vi "Deliver Result.vi"(8 "error in (no error)":errorcluster, 10 "result":refnum<class "result.lvclass">, 11 "input_poller_event in":refnum<class "input_poller_event.lvclass">) -> (0 "error out":errorcluster, 3 "input_poller_event out":refnum<class "input_poller_event.lvclass">)   [LabVIEW 2015, in "input_poller_event.lvclass"]
uses:
  input_poller_event.lvclass
  Result/result.lvclass
  input_poller_event.lvclass/input_poller_event.ctl
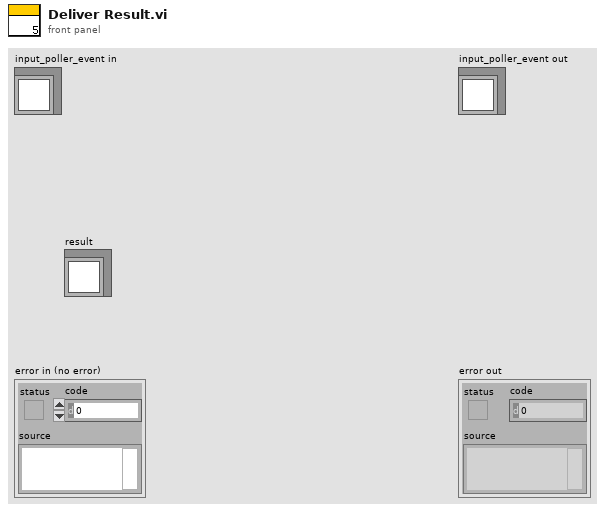
[diagram p1: front panel]
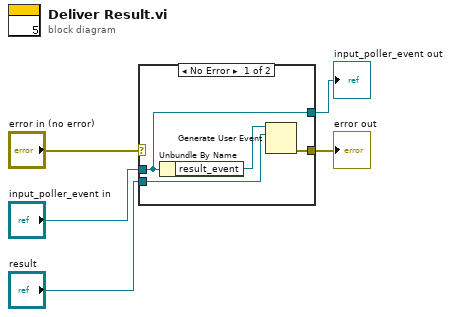
[diagram p0: block diagram]
diagram:
  n1 = case shown="No Error" "error in (no error)" {
    selector: "error in (no error)" -> [_ w11]
    tunnel: [w8 w11] -> w4
    tunnel: [w7 w10] -> w3
    tunnel: "input_poller_event in" -> [w7 w10]
    tunnel: "result" -> [w6 _]
    frame No Error {
      n2 = Unbundle By Name(w7) -> ("result_event"=w9:refnum<user-event>)
      n3 = Generate User Event(user event=w9, event data cluster=w6) -> (error out=w8:errorcluster)  [unwired: 2 in, 1 out]
    }
    frame Error {
    }
  }
  "error out" <- w4
  "input_poller_event out" <- w3
